vi "Unmarshal.vi"(8 "error in (no error)":errorcluster, 10 "Buffer":u8[](array[numeric]), 11 "Message in":refnum<class "Raw Message.lvclass">) -> (0 "error out":errorcluster, 2 "Buffer Count":i32=8, 3 "Message out":refnum<class "Raw Message.lvclass">)   [LabVIEW 2020, in "Protobuf RAW.lvlib" / "Raw Message.lvclass"]
uses:
  Raw Message.lvclass
  Raw Message.lvclass/Raw Message.ctl
  <vilib>/Utility/miscctls.llb/LVMapReplaceAction.ctl
  Tag/Basic Type.lvclass
  Protobuf RAW.lvlib
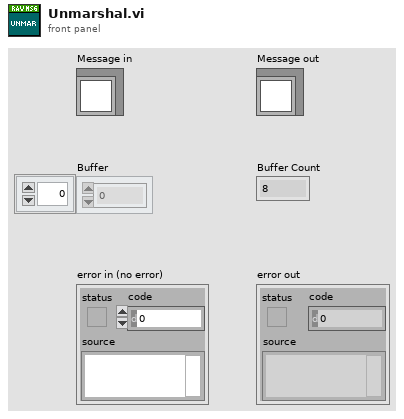
[diagram p1: front panel]
types:
  T1 = typedef "LVMapReplaceAction.ctl" = enum32{"Modify Entry only if found", "Add or Modify Entry", "Delete Entry"}
  T2 = typedef "Protobuf RAW.lvlib/Wire Chunk.ctl" = cluster{"ID":u32, "Wire Type":T3, "Buffer":u8[], "length":i32}
  T3 = typedef "Protobuf RAW.lvlib/Wire Type Group.lvclass/Wire Type.ctl" = enum16{"VARINT", "I64", "LEN", "SGROUP", "EGROUP", "I32"}
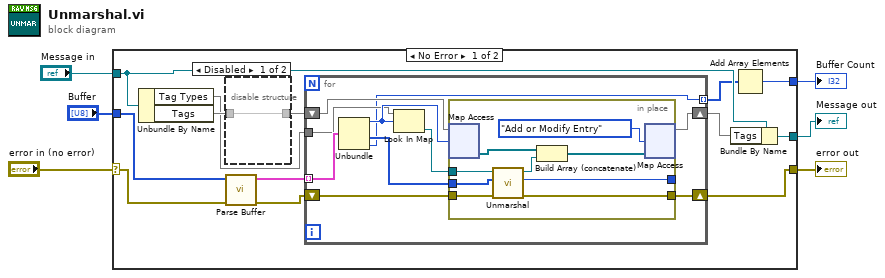
[diagram p0: block diagram]
diagram:
  n1 = case shown="No Error" "error in (no error)" {
    selector: "error in (no error)" -> [w17 w41]
    tunnel: "Message in" -> [w16 w40]
    tunnel: [w19 w40] -> w5
    tunnel: "Buffer" -> [w18 _]
    tunnel: [w10 w41] -> w3
    tunnel: [w8 _] -> w1
    frame No Error {
      n2 = Unbundle By Name(w16) -> ("Tag Types"=w14:map{u32, refnum<class "Basic Type.lvclass">}, "Tags"=w15:map{u32, refnum<class "Basic Type.lvclass">[]})
      n3 = disable-structure shown="Disabled" {
        disable-tunnel: [w39 _] -> w13
        disable-tunnel: w15 -> [w39 _]
        frame Disabled {
        }
        frame Enabled {
        }
      }
      n4 = call "Parse Buffer.vi"("error in (no error)"=w17, "Buffer"=w18) -> ("error out"=w12:errorcluster, "Raw Fields"=w7:T2[])  [unwired: 8 in]
      n5 = for {
        tunnel: w7 -> [w29] mode=indexing
        tunnel: w14 -> [w22]
        shift-right: [w26] -> w11
        shift-left: w13 -> [w27]
        shift-right: [w23] -> w10
        shift-left: w12 -> [w24]
        tunnel: [w20] -> w9 mode=indexing
        n6 = Unbundle(w29) -> ("ID"=w28:u32, "Buffer"=w25:u8[], "length"=w20:i32)  [unwired: 1 out]
        n7 = Look In Map(map=w22, key=w28) -> (value=w21:refnum<class "Basic Type.lvclass">)  [unwired: 1 in, 1 out]
        n8 = in-place {
          in-place-border: w24 -> [w38]
          in-place-border: w25 -> [w37]
          in-place-border: [w36] -> w23
          in-place-border: w21 -> [w31]
          in-place-border: [w30] -> _
          n9 = in-place-map #1(w27, w28) -> (w35:refnum<class "Basic Type.lvclass">[])  [unwired: 1 in, 1 out]
          n10 = call-dynamic "Unmarshal.vi"("error in (no error)"=w38, "Buffer"=w37, "Tag in"=w31) -> ("error out"=w36:errorcluster, "Buffer Count"=w30:i32, "Tag out"=w33:refnum<class "Basic Type.lvclass">)  [unwired: 6 in]
          n11 = Build Array (concatenate)(w35, w33) -> (w34:refnum<class "Basic Type.lvclass">[])
          n12 = in-place-map #1(w34, LVMapReplaceAction."Add or Modify Entry" ("action")) -> (w26:map{u32, refnum<class "Basic Type.lvclass">[]})  [unwired: 2 out]
        }
      }
      n13 = Bundle By Name(cluster=w16, "Tags"=w11) -> (w19:refnum<class "Raw Message.lvclass">)
      n14 = Add Array Elements(numeric array=w9) -> (sum=w8:i32)
    }
    frame Error {
    }
  }
  "error out" <- w3
  "Message out" <- w5
  "Buffer Count" <- w1
